vi "Create All Message Queues.vi"(8 "error in (no error)":errorcluster, 11 "Process Name":string) -> (0 "error out":errorcluster, 3 "Message Queues":T1)   [LabVIEW 2018, in "D-O Module.lvlib"]
uses:
  D-O Module.lvlib
  All Message Queues.ctl
  support/Message Queue/Message Cluster.ctl
  D-O Module Settings Cluster.ctl
  D-O Device Settings Cluster.ctl
  VICI Electronic Actuator/VICI Electronic Actuator Settings.ctl
  support/Message Queue/Enqueue Message (Single).vi
  support/Message Queue/Message Queue.lvlib
  DIO Valve/VICI Electronic Actuator.lvlib
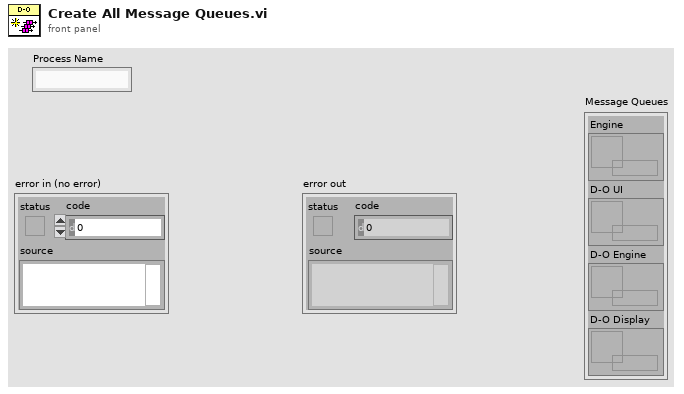
[diagram p1: front panel]
types:
  T1 = typedef "D-O Module.lvlib/All Message Queues.ctl" = cluster{"Engine":refnum<queue>, "D-O UI":refnum<queue>, "D-O Engine":refnum<queue>, "D-O Display":refnum<queue>}
  T2 = typedef "D-O Module.lvlib/D-O Module Settings Cluster.ctl" = cluster{"D-O Settings":T3, "VICI Electronic Actuator":T4}
  T3 = typedef "D-O Module.lvlib/D-O Device Settings Cluster.ctl" = cluster{"DAQmx Task Name":refnum<k21>, "Output Channel":u16, "Output Channel Names":string[]}
  T4 = typedef "VICI Electronic Actuator.lvlib/VICI Electronic Actuator Settings.ctl" = cluster{"VISA resource name":refnum<visa-resource-name>, "Mode":enum16{"Two Positions With Stops", "Two Positions Without Stops", "Mutiposition"}, "Simulated":bool}
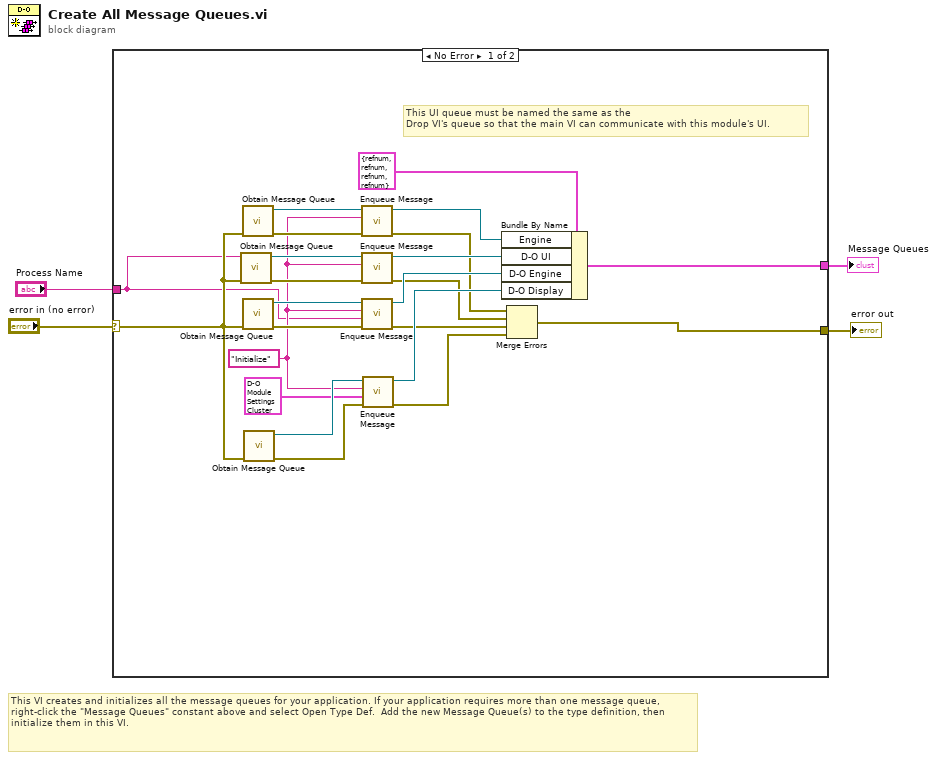
[diagram p0: block diagram]
diagram:
  # "This VI creates and initializes all the message queues for your application. If your application requires more than one message queue, right-click the \"Message Queues\" constant above and select Open Type Def.  Add the new Message Queue(s) to the type definition, then initialize them in this VI."
  n1 = case shown="No Error" "error in (no error)" {
    selector: "error in (no error)" -> [w13 w28]
    tunnel: [w26 w28] -> w4
    tunnel: [w27 _] -> w2
    tunnel: "Process Name" -> [w5 _]
    frame No Error {
      w6 = "Initialize" ("Message")
      # "This UI queue must be named the same as the \nDrop VI's queue so that the main VI can communicate with this module's UI."
      n2 = call "Obtain Message Queue.vi"("error in (no error)"=w13, "name (unnamed)"=w5) -> ("error out"=w14:errorcluster, "Message Queue"=w22:refnum<queue>)  [unwired: 8 in]
      n3 = call "Obtain Message Queue.vi"("error in (no error)"=w13) -> ("error out"=w24:errorcluster, "Message Queue"=w25:refnum<queue>)  [unwired: 9 in]
      n4 = call "Obtain Message Queue.vi"("error in (no error)"=w13) -> ("error out"=w20:errorcluster, "Message Queue"=w21:refnum<queue>)  [unwired: 9 in]
      n5 = call "Obtain Message Queue.vi"("error in (no error)"=w13) -> ("error out"=w18:errorcluster, "Message Queue"=w19:refnum<queue>)  [unwired: 9 in]
      n6 = call-poly "Enqueue Message.vi"("error in (no error)"=w24, "Message"=w6, "Message Queue"=w25) -> ("error out"=w11:errorcluster, "dup Message Queue"=w23:refnum<queue>)  [unwired: 7 in]
      n7 = call-poly "Enqueue Message.vi"("error in (no error)"=w14, "Message"=w6, "Message Queue"=w22) -> ("error out"=w9:errorcluster, "dup Message Queue"=w17:refnum<queue>)  [unwired: 7 in]
      n8 = call-poly "Enqueue Message.vi"("error in (no error)"=w20, "Message Data"=w5, "Message"=w6, "Message Queue"=w21) -> ("error out"=w10:errorcluster, "dup Message Queue"=w16:refnum<queue>)  [unwired: 6 in]
      n9 = call-poly "Enqueue Message.vi"("error in (no error)"=w18, "Message Data"=T2 {"D-O Settings"={"DAQmx Task Name"="", "Output Channel"=0, "Output Channel Names"=[]}, "VICI Electronic Actuator"={"VISA resource name"="", "Mode"=enum."Two Positions With Stops", "Simulated"=FALSE}} ("D-O Configuration"), "Message"=w6, "Message Queue"=w19) -> ("error out"=w7:errorcluster, "dup Message Queue"=w15:refnum<queue>)  [unwired: 6 in]
      n10 = Bundle By Name(cluster=T1 {"Engine"=refnum, "D-O UI"=refnum, "D-O Engine"=refnum, "D-O Display"=refnum} ("Message Queues"), "Engine"=w23, "D-O UI"=w17, "D-O Engine"=w16, "D-O Display"=w15) -> (w27:T1)
      n11 = Merge Errors(w11, w9, w10, w7) -> (w26:errorcluster)
    }
    frame Error {
    }
  }
  "Message Queues" <- w2
  "error out" <- w4
